vi "Create.vi"(10 "Status ref":refnum<vi>, 11 "Paths":T1={"ComicRootPath"=path "C:/data/comics/comics", "SeriesRootPath"=path "C:/data/comics/series", "WeeklyRootPath"=path "C:/data/comics/weeklies", "CharacterRootPath"=path "C:/data/comics/characters", "CreatorRootPath"=path "C:/data/comics/creators", "CachePath"=path "C:/data/comics/cache"}) -> (3 "Comics.lvclass":refnum<class "Comics.lvclass">)   [LabVIEW 2022 SP3, in "Comics.lvclass"]
uses:
  Comics.lvclass
  TypeDefs/Paths.ctl
  Comics.lvclass/Comics.ctl
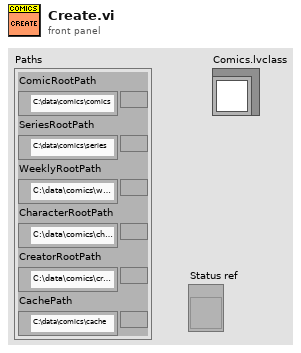
[diagram p1: front panel]
types:
  T1 = typedef "Paths.ctl" = cluster{"ComicRootPath":path, "SeriesRootPath":path, "WeeklyRootPath":path, "CharacterRootPath":path, "CreatorRootPath":path, "CachePath":path}
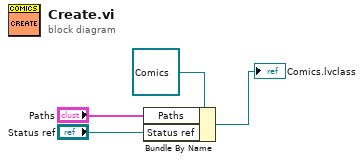
[diagram p0: block diagram]
diagram:
  n1 = Bundle By Name(cluster=refnum<class "Comics.lvclass"> refnum ("Comics.lvclass"), "Paths"="Paths", "Status ref"="Status ref") -> (→"Comics.lvclass":refnum<class "Comics.lvclass">)
